vi "Burning2.1.vi"() -> ()   [LabVIEW 2022 SP3]
uses:
  Loop Handler/Main/Type Def/MainStates Cluster.ctl
  Loop Handler/Main/Type Def/MainStates.ctl
panel:
  out "Cartucho 8":dbl(graph)
  out "Cartucho 7":dbl(graph)
  out "Cartucho 6":dbl(graph)
  out "Cartucho 5":dbl(graph)
  out "Cartucho 4":dbl(graph)
  out "Cartucho 3":dbl(graph)
  out "Cartucho 2":dbl(graph)
  out "Cartucho 1":dbl(graph)
  out "0":cluster{i32, i32, i32, i32, i32, i32, i32, i32}={0, 1, 4, 5, 6, 7, 2, 3}
  out "Array":dbl[](array[numeric])
  in  "Cluster":T1
  in  "Prueba C":T2
  in  "SettingsCluster":T3={"OK Button Settings"=FALSE, "Default Set"=FALSE, "D Turbine"=FALSE, "D Panel"=FALSE, "D Date"=FALSE, "Delete Results"=FALSE, "file"=path "D:/config.ini"}
  out "Done":bool
  out "Start Time":string
  out "End Time":string
  out "Current Time":string
  out "Tmin":dbl
  out "Tmax":dbl
  out "CoolD":dbl
  out "TestT":dbl
  out "Contra":string
  out "values":string[](array[string])
  in  "Stop Test":bool
  in  "Start Test":bool
  in  "String 2":string
  out "Boolean":bool
  out "Numeric 2":dbl
  out "Array 3":string[](array[string])
  in  "Part Number":string
  in  "Help":bool
  out "EMO":bool
  in  "Cartuchos":u32[](array[colorbox]) caption="Cartridges"
  in  "Settings":bool
  in  "Results":bool
  in  "U settings":bool
  in  "Exit Button":bool
  in  "Lenguage":bool
  in  "Sets":T4
  out "offset past number":i32
  out "number":dbl
  out "data out":string
  out "bytes written":i32
  out "Numeric":dbl
  out "date/time string":string
  out "Acción":string
  out "Voltaje de salida":dbl caption="Output Voltage"
  in  "Voltage":bool
  in  "Probes":bool
  out "No. T":dbl caption="No. of Tests"
  out "Indicators":T5={"Error Out Array"=[], "Modbus"=FALSE, "Enet"=FALSE, "Ready"=FALSE, "Voltage output"=FALSE, "Prueba"=TRUE}
  # "MSE"
  # "1"
  # "2"
  # "3"
  # "4"
  # "5"
  # "6"
  # "7"
  # "8"
  # "DC Voltage"
  # "AC Voltage"
  # "Test"
  # "SETTINGS"
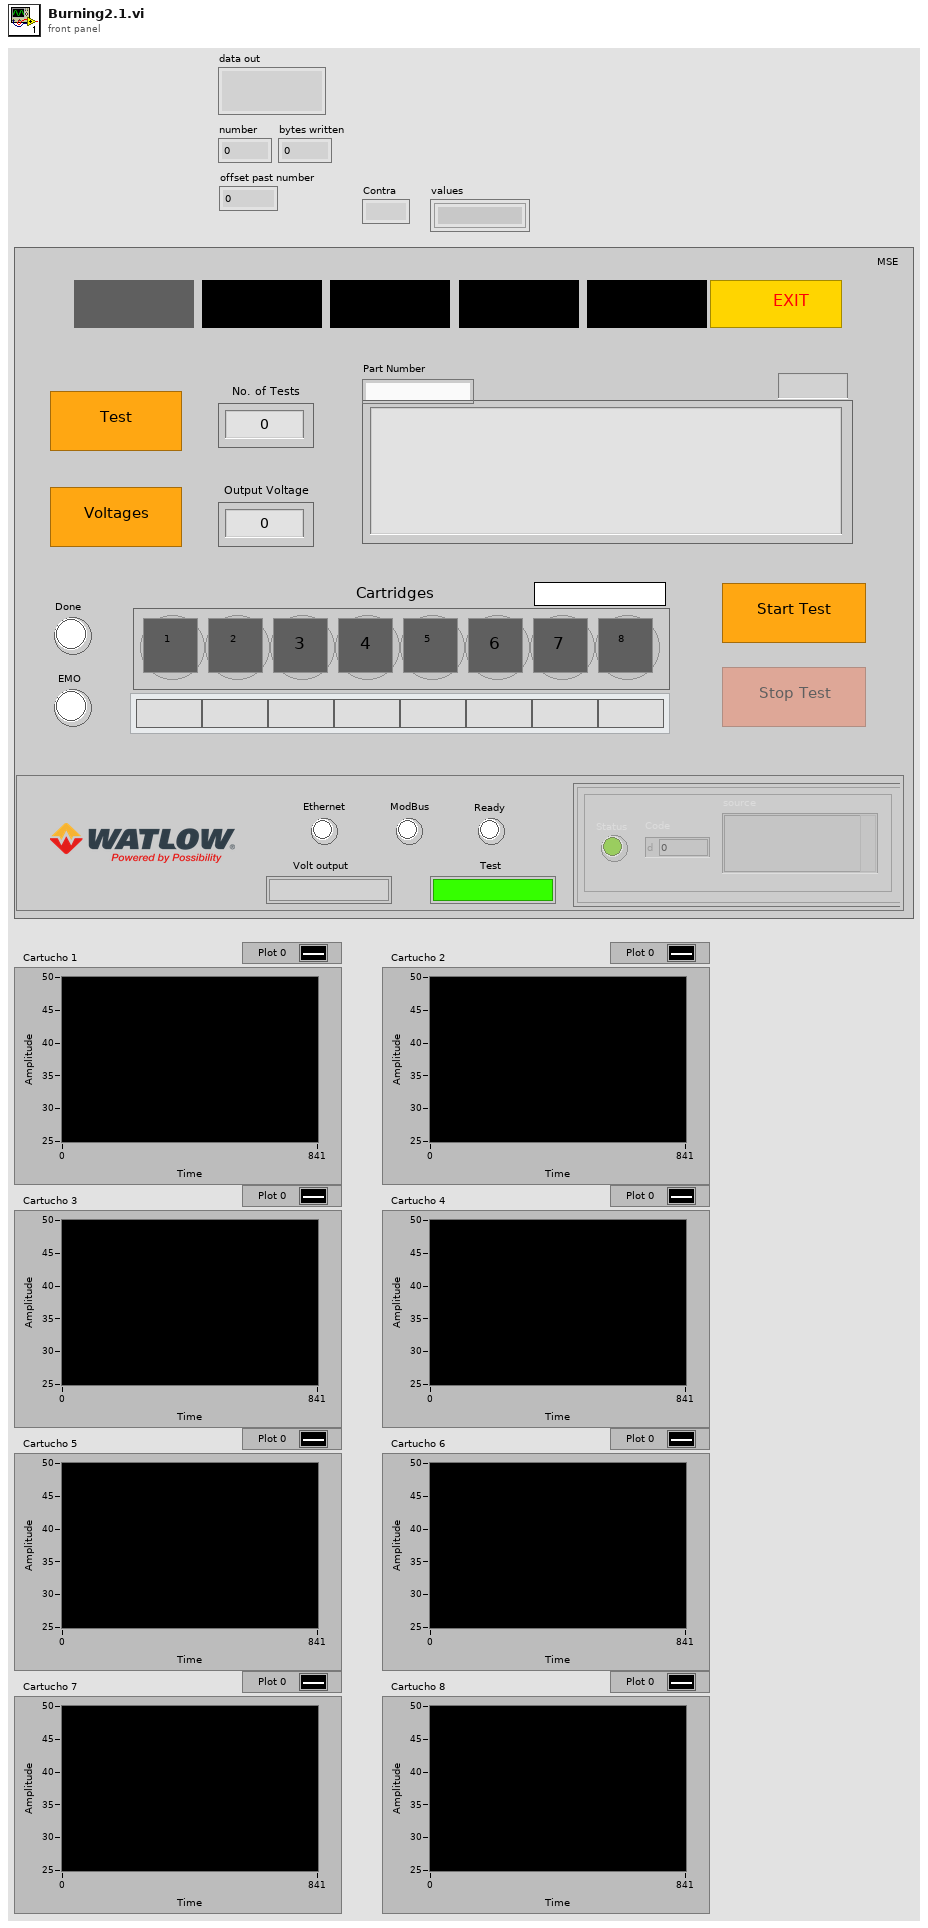
[diagram p1: front panel]
types:
  T1 = cluster{"24v":bool, "48v":bool, "110v":bool, "220v":bool, "OK Button Volts":bool, "Cancel Button Volts":bool}
  T2 = cluster{"OK Button":bool, "Tiempo Prueba":dbl, "Tiempo enfriamiento":dbl, "Temp- Max":dbl, "Tempo - Min":dbl, "Default Test":bool, "Cancel Button Test":bool}
  T3 = cluster{"OK Button Settings":bool, "Default Set":bool, "D Turbine":bool, "D Panel":bool, "D Date":bool, "Delete Results":bool, "file":path}
  T4 = cluster{"String":string, "String 2":string, "String 3":string, "String 4":string}
  T5 = cluster{"Error Out Array":errorcluster[], "Modbus":bool, "Enet":bool, "Ready":bool, "Voltage output":bool, "Prueba":bool}
  T6 = typedef "MainStates Cluster.ctl" = cluster{"States":T7, "Data":variant}
  T7 = typedef "MainStates.ctl" = enum16{"Open Ports", "Set_Config", "Close Ports", "Main", "Settings", "Volts", "Lenguaje", "Test", "End test", "EMO", "Exit"}
  T8 = cluster{"Error Out Array":errorcluster[], "34970A":bool, "53220A":bool, "USB-CAN":bool, "USB-LIN":bool, "Voltage output":bool}
  T9 = enum8{"Enabled", "Disabled", "Disabled and Grayed Out"}
  T10 = enum16{"Standard", "Buffered", "CRLF", "Immediate"}
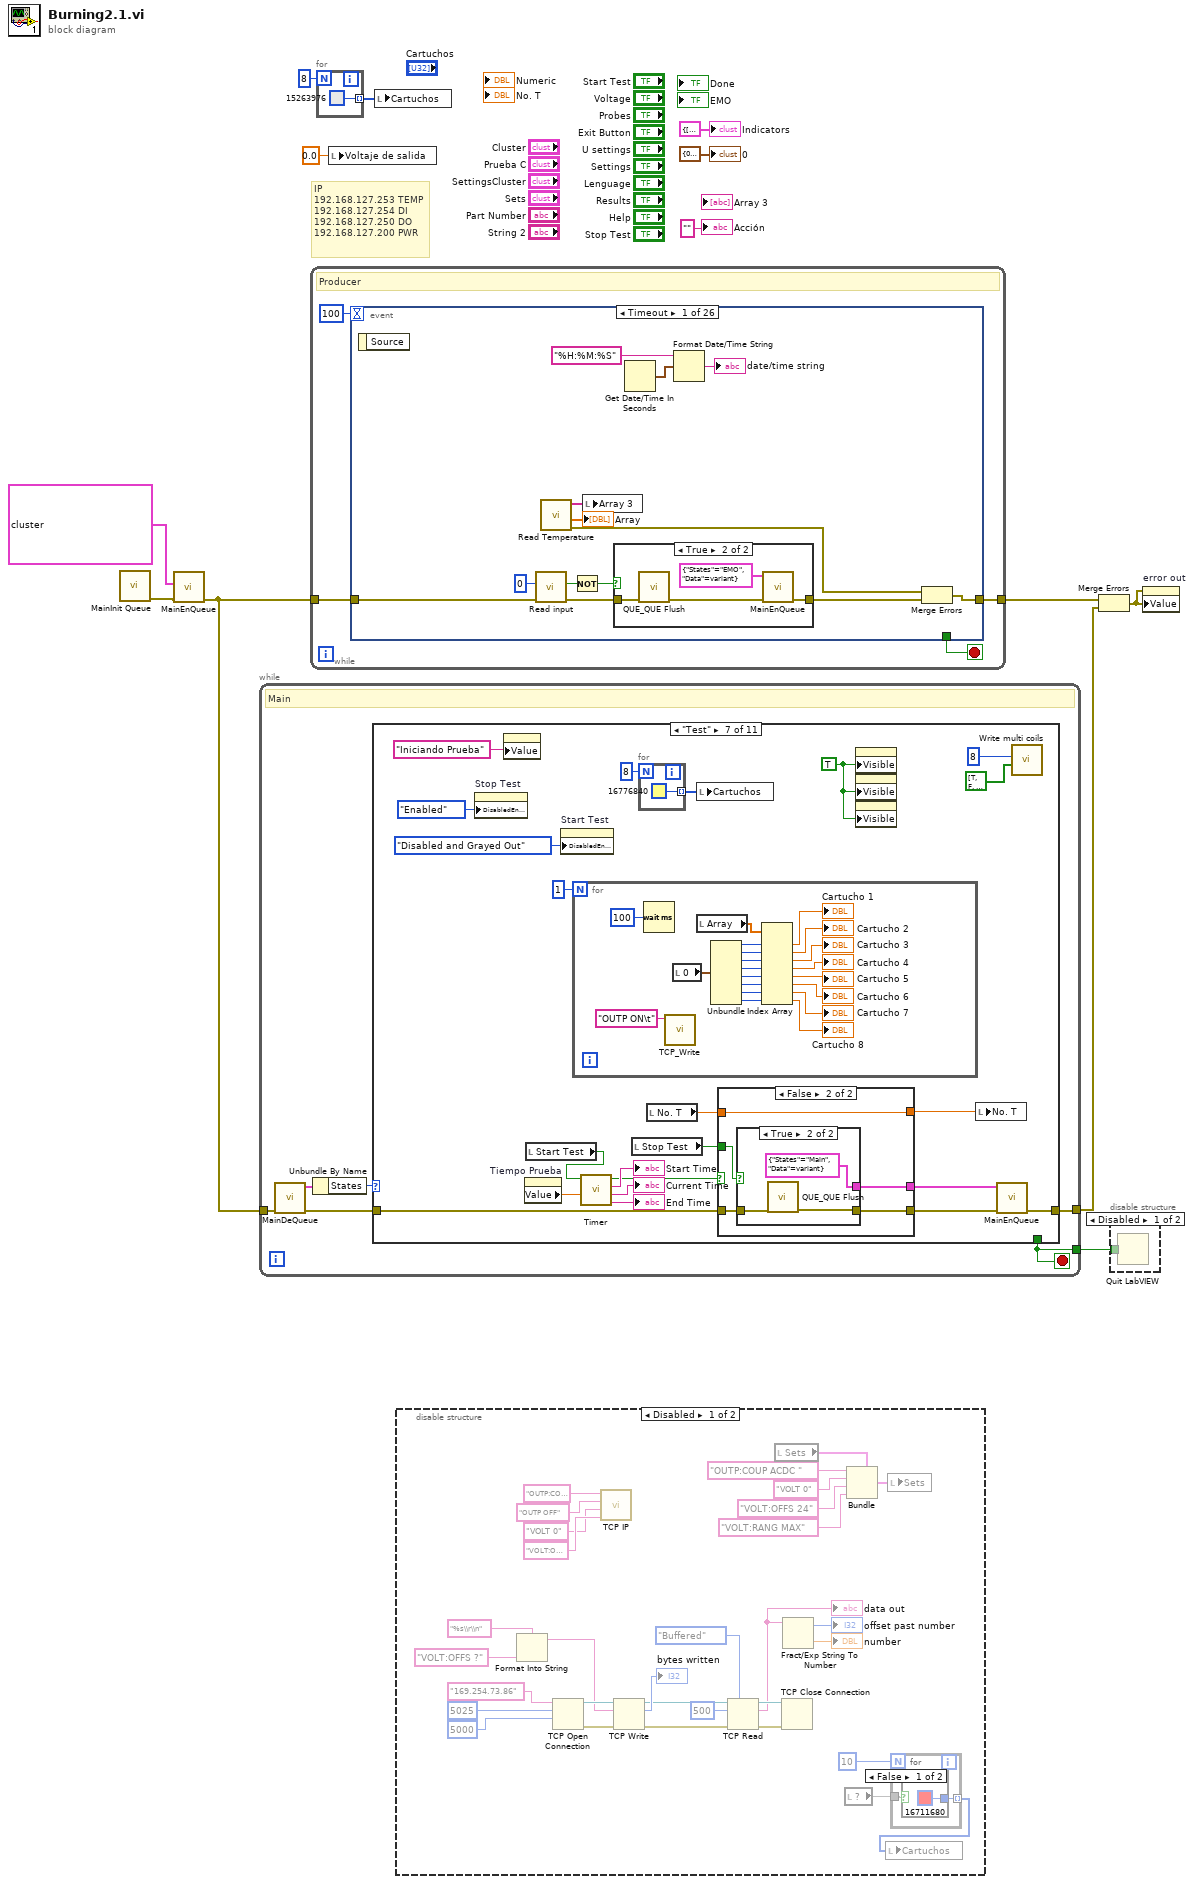
[diagram p0: block diagram]
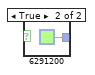
[diagram p2: hidden frame]
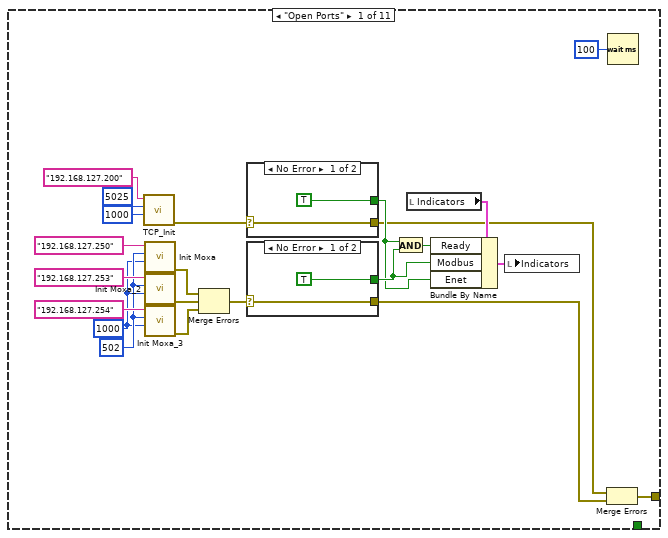
[diagram p5: hidden frame]
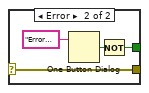
[diagram p6: hidden frame]
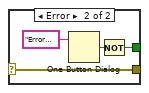
[diagram p7: hidden frame]
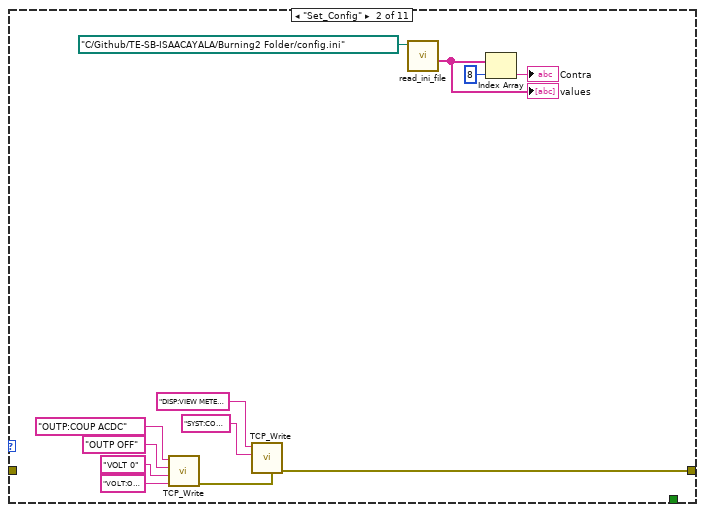
[diagram p8: hidden frame]
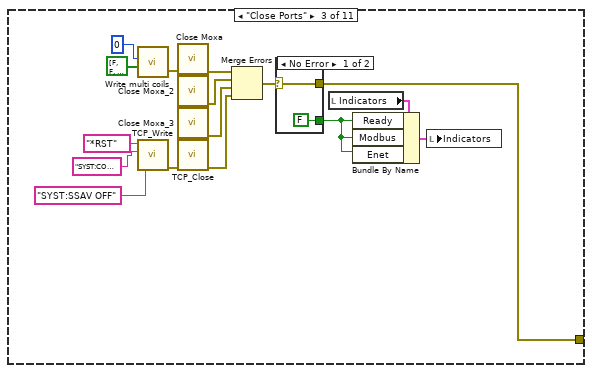
[diagram p9: hidden frame]
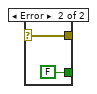
[diagram p10: hidden frame]
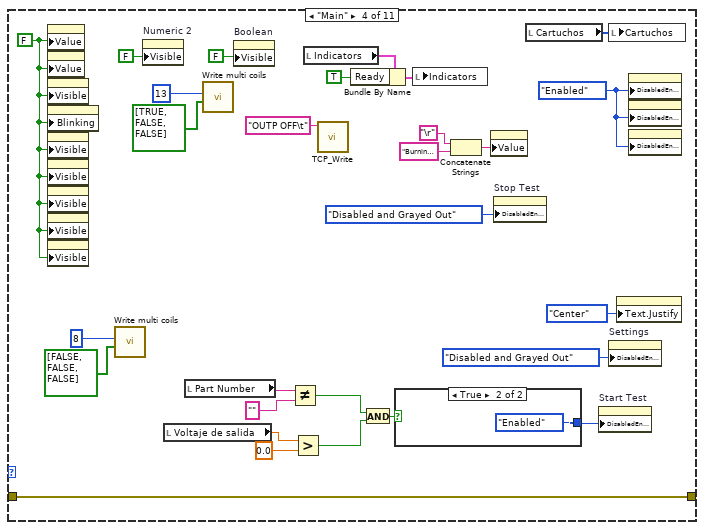
[diagram p11: hidden frame]
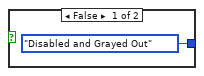
[diagram p12: hidden frame]
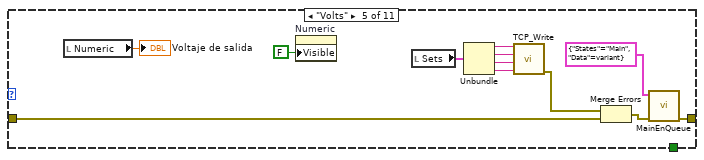
[diagram p13: hidden frame]
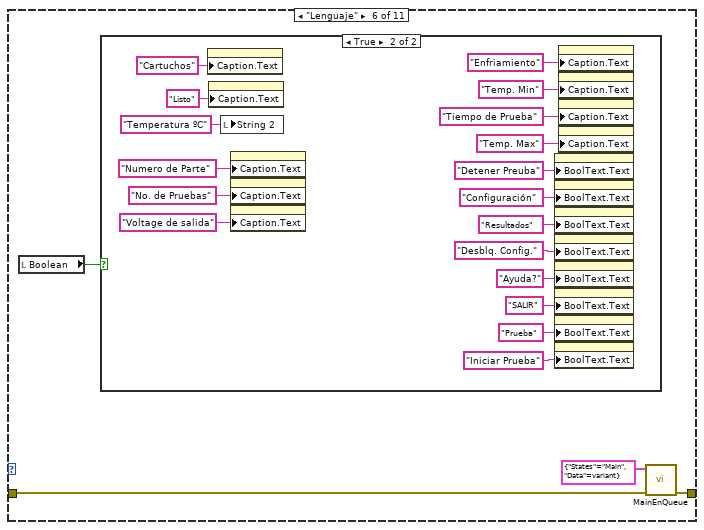
[diagram p14: hidden frame]
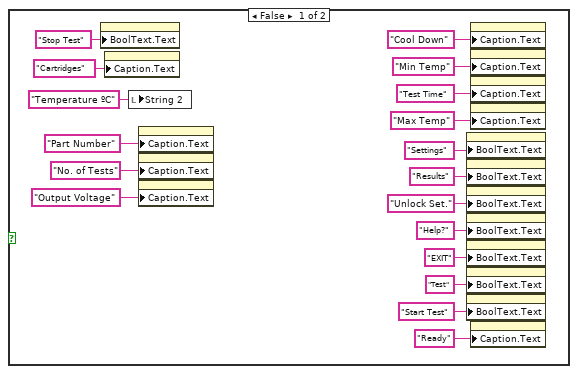
[diagram p15: hidden frame]
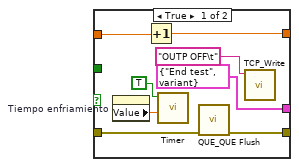
[diagram p16: hidden frame]
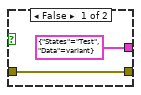
[diagram p17: hidden frame]
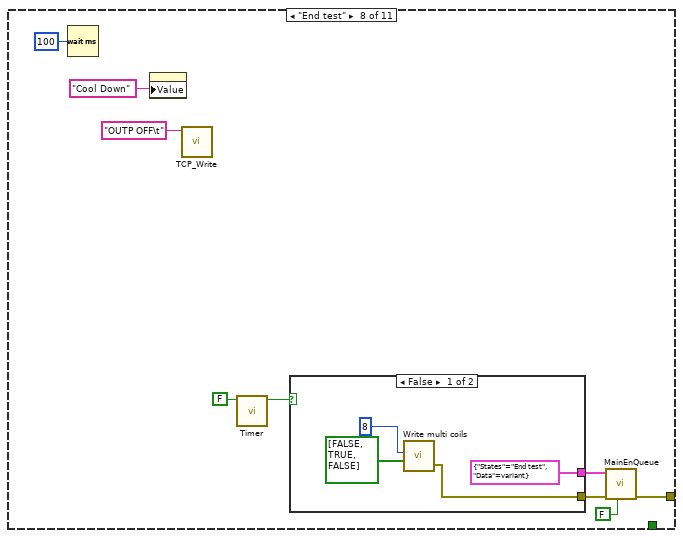
[diagram p18: hidden frame]
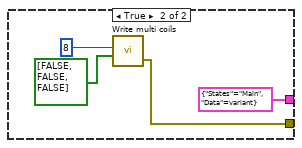
[diagram p19: hidden frame]
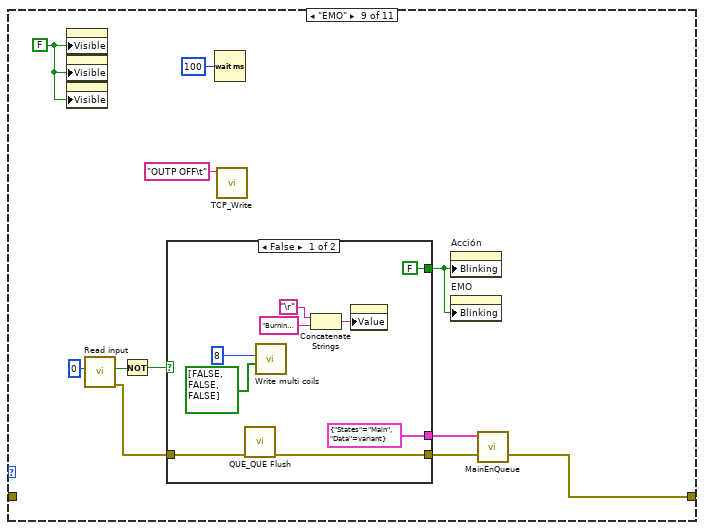
[diagram p20: hidden frame]
diagram:
  # "IP\n192.168.127.253 TEMP\n192.168.127.254 DI\n192.168.127.250 DO \n192.168.127.200 PWR"
  n1 = call "MainInit Queue.vi"() -> ("error out"=w11:errorcluster)  [unwired: 11 in]
  n2 = call "MainEnQueue.vi"("error in"=w11, "Array States"=T6[] [{"States"=enum."Open Ports", "Data"=variant}, {"States"=enum."Set_Config", "Data"=variant}, {"States"=enum."Main", "Data"=variant}]) -> ("error out"=w10:errorcluster)  [unwired: 9 in]
  n3 = while {
    tunnel: [w19] -> w8
    tunnel: [w18] -> w13
    tunnel: w10 -> [w16]
    stop <- w18 stop-if-true
    # "Main"
    n4 = call "MainDeQueue.vi"("error in"=w16) -> ("error out"=w15:errorcluster, "States"=w17:T6)  [unwired: 8 in, 1 out]
    n5 = Unbundle By Name(w17) -> ("States"=w14:T7)
    n6 = case shown="\"Test\"" w14 {
      tunnel: [_ _ _ _ _ _ _ _ _ TRUE _] -> w18
      tunnel: [w22 w58 w74 w90 w127 w131 w172 w237 w252 w276 _] -> w19
      tunnel: w15 -> [_ _ _ w90 w118 w128 w175 _ _ _ _]
      frame "Open Ports" {
        w30 = 1000 ("connect timeout ms")
        w31 = u16 502 ("port")
        n7 = call "TCP_Init.vi"("timeout ms (60000)"=1000, "remote port or service name"=u16 5025, "address"="192.168.127.200") -> ("error out 2"=w26:errorcluster)  [unwired: 6 in, 2 out]
        n8 = call "Init Moxa.vi"("connect timeout ms"=w30, "port"=w31, "Address"="192.168.127.250") -> ("error out"=w34:errorcluster)  [unwired: 6 in, 2 out]
        n9 = call "Init Moxa_2.vi"("connect timeout ms"=w30, "port"=w31, "Address"="192.168.127.253") -> ("error out"=w33:errorcluster)  [unwired: 6 in, 2 out]
        n10 = call "Init Moxa_3.vi"("connect timeout ms"=w30, "port"=w31, "Address"="192.168.127.254") -> ("error out"=w32:errorcluster)  [unwired: 6 in, 2 out]
        n11 = Merge Errors(w34, w33, w32) -> (w41:errorcluster)
        n12 = case shown="No Error" w26 {
          selector: w26 -> [w43 w46]
          tunnel: [w43 w46] -> w21
          tunnel: [TRUE ("true") w45] -> w23
          frame No Error {
          }
          frame Error {
            n13 = One Button Dialog(message="Error Power Supply") -> (true=w44:bool)  [unwired: 1 in]
            n14 = Not(x=w44) -> (.not. x?=w45:bool)
          }
        }
        n15 = case shown="No Error" w41 {
          selector: w41 -> [w49 w52]
          tunnel: [w49 w52] -> w20
          tunnel: [TRUE ("true") w51] -> w24
          frame No Error {
          }
          frame Error {
            n16 = One Button Dialog(message="Error Moxas") -> (true=w50:bool)  [unwired: 1 in]
            n17 = Not(x=w50) -> (.not. x?=w51:bool)
          }
        }
        n18 = And(x=w23, y=w24) -> (x .and. y?=w25:bool)
        n19 = local read "Indicators"() -> (w40:T5)
        n20 = Bundle By Name(cluster=w40, "Ready"=w25, "Modbus"=w24, "Enet"=w23) -> (w39:T5)
        n21 = local write "Indicators"(w39) -> ()
        n22 = Merge Errors(w21, w20) -> (w22:errorcluster)
        n23 = Wait (ms)(milliseconds to wait=u32 100) -> ()  [unwired: 1 out]
      }
      frame "Set_Config" {
        n24 = call "TCP_Write.vi"("String 1"="OUTP:COUP ACDC", "String 4"="OUTP OFF" ("String 2"), "String 3"="VOLT 0", "String 2"="VOLT:OFFS 0" ("String 4")) -> ("error out"=w61:errorcluster)  [unwired: 4 in, 1 out]
        n25 = call "TCP_Write.vi"("String 1"="DISP:VIEW METER_VI\n", "String 4"="SYST:COMM:RLST RWL", "error in (no error) 2"=w61) -> ("error out"=w58:errorcluster)  [unwired: 5 in, 1 out]
        n26 = call "read_ini_file.vi"("configuration file path"=path "C:/Github/TE-SB-ISAACAYALA/Burning2 Folder/config.ini") -> ("values"=w56:string[])  [unwired: 7 in, 3 out]
        "values" <- w56
        n27 = Index Array(array=w56, index=8) -> (element=→"Contra":string)
      }
      frame "Close Ports" {
        n28 = call "Write multi coils.vi"("coils to write"=bool[] [FALSE, FALSE, FALSE, FALSE, FALSE, FALSE, FALSE, FALSE, FALSE, FALSE, FALSE, FALSE, FALSE, FALSE, FALSE], "starting address"=u16 0) -> ("error IO"=w71:errorcluster)  [unwired: 2 in, 1 out]
        n29 = call "TCP_Write.vi"("String 1"="*RST", "String 4"="SYST:COMM:RLST LOC", "String 3"="SYST:SSAV OFF") -> ("error out"=w68:errorcluster)  [unwired: 5 in, 1 out]
        n30 = call "Close Moxa.vi"("error in (no error)"=w71) -> ("error out"=w79:errorcluster)  [unwired: 10 in]
        n31 = call "Close Moxa_2.vi"() -> ("error out"=w80:errorcluster)  [unwired: 11 in]
        n32 = call "Close Moxa_3.vi"() -> ("error out"=w81:errorcluster)  [unwired: 11 in]
        n33 = call "TCP_Close.vi"("error in (no error) 2"=w68) -> ("error out"=w70:errorcluster)  [unwired: 10 in]
        n34 = Merge Errors(w79, w80, w81, w70) -> (w76:errorcluster)
        n35 = case shown="No Error" w76 {
          selector: w76 -> [w82 w85]
          tunnel: [FALSE ("Enet") FALSE ("Enet")] -> w75
          tunnel: [w82 w85] -> w74
          frame No Error {
          }
          frame Error {
          }
        }
        n36 = local read "Indicators"() -> (w78:T5)
        n37 = Bundle By Name(cluster=w78, "Ready"=w75, "Modbus"=w75, "Enet"=w75) -> (w77:T5)
        n38 = local write "Indicators"(w77) -> ()
      }
      frame "Main" {
        w87 = FALSE ("Value")
        w107 = T9."Enabled" ("Disabled")
        n39 = property on="Prueba" class="Bool (strict)"("Value"=w87) -> ()  [unwired: 2 in, 2 out]
        n40 = property on="Voltage output" class="Bool (strict)"("Value"=w87) -> ()  [unwired: 2 in, 2 out]
        n41 = property on="SettingsCluster" class="Clust (strict)"("Visible"=w87) -> ()  [unwired: 2 in, 2 out]
        n42 = property on="Acción" class="Str"("Blinking"=w87) -> ()  [unwired: 2 in, 2 out]
        n43 = property on="Cluster" class="Clust (strict)"("Visible"=w87) -> ()  [unwired: 2 in, 2 out]
        n44 = property on="Prueba C" class="Clust (strict)"("Visible"=w87) -> ()  [unwired: 2 in, 2 out]
        n45 = property on="Start Time" class="Str"("Visible"=w87) -> ()  [unwired: 2 in, 2 out]
        n46 = property on="End Time" class="Str"("Visible"=w87) -> ()  [unwired: 2 in, 2 out]
        n47 = property on="Current Time" class="Str"("Visible"=w87) -> ()  [unwired: 2 in, 2 out]
        n48 = call "Write multi coils.vi"("coils to write"=bool[] [FALSE, FALSE, FALSE], "starting address"=u16 8) -> ()  [unwired: 2 in, 2 out]
        n49 = property on="Numeric 2" class="DigNum (strict)"("Visible"=FALSE) -> ()  [unwired: 2 in, 2 out]
        n50 = local read "Voltaje de salida"() -> (w100:dbl)
        n51 = local read "Part Number"() -> (w98:string)
        n52 = call "Write multi coils.vi"("coils to write"=bool[] [TRUE, FALSE, FALSE], "starting address"=u16 13) -> ()  [unwired: 2 in, 2 out]
        n53 = property on="Boolean" class="Bool (strict)"("Visible"=FALSE) -> ()  [unwired: 2 in, 2 out]
        n54 = Not Equal?(x=w98, y="") -> (x != y?=w95:bool)
        n55 = Greater?(x=w100, y=0.0 ("x")) -> (0:w96:bool)
        n56 = local read "Indicators"() -> (w111:T5)
        n57 = call "TCP_Write.vi"("String 1"="OUTP OFF\t") -> ()  [unwired: 7 in, 2 out]
        n58 = Bundle By Name(cluster=w111, "Ready"=TRUE) -> (w110:T5)
        n59 = And(x=w95, y=w96) -> (x .and. y?=w94:bool)
        n60 = case shown="True" w94 {
          tunnel: [T9."Disabled and Grayed Out" ("Disabled") T9."Enabled" ("Disabled")] -> w101
          frame False {
          }
          frame True {
          }
        }
        n61 = local write "Indicators"(w110) -> ()
        n62 = Concatenate Strings("\r" ("Carriage Return Constant"), "Burning Tester 1.1" ("Acción")) -> (w106:string)
        n63 = property on="Acción" class="Str"("Value"=w106) -> ()  [unwired: 2 in, 2 out]
        n64 = property on="Stop Test" class="Bool (strict)"("DisabledEnum"=T9."Disabled and Grayed Out" ("Disabled")) -> ()  [unwired: 2 in, 2 out]
        n65 = local read "Cartuchos"() -> (w113:u32[])
        n66 = property on="Start Test" class="Bool (strict)"("DisabledEnum"=w101) -> ()  [unwired: 2 in, 2 out]
        n67 = local write "Cartuchos"(w113) -> ()
        n68 = property on="Settings" class="Bool (strict)"("DisabledEnum"=T9."Disabled and Grayed Out" ("Disabled")) -> ()  [unwired: 2 in, 2 out]
        n69 = property on="Acción" class="Str"("Text.Justify"=enum16{"Left", "Center", "Right"}."Center" ("Text.Justification")) -> ()  [unwired: 2 in, 2 out]
        n70 = property on="Voltage" class="Bool (strict)"("DisabledEnum"=w107) -> ()  [unwired: 2 in, 2 out]
        n71 = property on="Probes" class="Bool (strict)"("DisabledEnum"=w107) -> ()  [unwired: 2 in, 2 out]
        n72 = property on="U settings" class="Bool (strict)"("DisabledEnum"=w107) -> ()  [unwired: 2 in, 2 out]
      }
      frame "Volts" {
        n73 = local read "Numeric"() -> (→"Voltaje de salida":dbl)
        n74 = property on="Numeric" class="DigNum (strict)"("Visible"=FALSE) -> ()  [unwired: 2 in, 2 out]
        n75 = local read "Sets"() -> (w124:T4)
        n76 = Unbundle(w124) -> ("String"=w122:string, "String 2"=w121:string, "String 3"=w120:string, "String 4"=w119:string)
        n77 = call "TCP_Write.vi"("String 1"=w122, "String 4"=w121, "String 3"=w120, "String 2"=w119) -> ("error out"=w117:errorcluster)  [unwired: 4 in, 1 out]
        n78 = Merge Errors(w117, w118) -> (w116:errorcluster)
        n79 = call "MainEnQueue.vi"("error in"=w116, "States"=T6 {"States"=enum."Main", "Data"=variant}) -> ("error out"=w127:errorcluster)  [unwired: 9 in]
      }
      frame "Lenguaje" {
        n80 = local read "Boolean"() -> (w129:bool)
        n81 = case shown="True" w129 {
          frame False {
            n82 = property on="Stop Test" class="Bool (strict)"("BoolText.Text"="Stop Test" ("Boolean Text.Text")) -> ()  [unwired: 2 in, 2 out]
            n83 = property on="Cartuchos" class="Arr (strict)"("Caption.Text"="Cartridges") -> ()  [unwired: 2 in, 2 out]
            n84 = local write "String 2"("Temperature ºC" ("String 2")) -> ()
            n85 = property on="Part Number" class="Str"("Caption.Text"="Part Number") -> ()  [unwired: 2 in, 2 out]
            n86 = property on="No. T" class="DigNum (strict)"("Caption.Text"="No. of Tests") -> ()  [unwired: 2 in, 2 out]
            n87 = property on="Voltaje de salida" class="DigNum (strict)"("Caption.Text"="Output Voltage") -> ()  [unwired: 2 in, 2 out]
            n88 = property on="Settings" class="Bool (strict)"("BoolText.Text"="Settings" ("Boolean Text.Text")) -> ()  [unwired: 2 in, 2 out]
            n89 = property on="Results" class="Bool (strict)"("BoolText.Text"="Results" ("Boolean Text.Text")) -> ()  [unwired: 2 in, 2 out]
            n90 = property on="U settings" class="Bool (strict)"("BoolText.Text"="Unlock Set." ("Boolean Text.Text")) -> ()  [unwired: 2 in, 2 out]
            n91 = property on="Help" class="Bool (strict)"("BoolText.Text"="Help?" ("Boolean Text.Text")) -> ()  [unwired: 2 in, 2 out]
            n92 = property on="Exit Button" class="Bool (strict)"("BoolText.Text"="EXIT" ("Boolean Text.Text")) -> ()  [unwired: 2 in, 2 out]
            n93 = property on="Probes" class="Bool (strict)"("BoolText.Text"="Test" ("Boolean Text.Text")) -> ()  [unwired: 2 in, 2 out]
            n94 = property on="Start Test" class="Bool (strict)"("BoolText.Text"="Start Test" ("Boolean Text.Text")) -> ()  [unwired: 2 in, 2 out]
            n95 = property on="Tiempo enfriamiento" class="DigNum (strict)"("Caption.Text"="Cool Down") -> ()  [unwired: 2 in, 2 out]
            n96 = property on="Tempo - Min" class="DigNum (strict)"("Caption.Text"="Min Temp") -> ()  [unwired: 2 in, 2 out]
            n97 = property on="Tiempo Prueba" class="DigNum (strict)"("Caption.Text"="Test Time") -> ()  [unwired: 2 in, 2 out]
            n98 = property on="Temp- Max" class="DigNum (strict)"("Caption.Text"="Max Temp") -> ()  [unwired: 2 in, 2 out]
            n99 = property on="Ready" class="Bool (strict)"("Caption.Text"="Ready") -> ()  [unwired: 2 in, 2 out]
          }
          frame True {
            n100 = property on="Cartuchos" class="Arr (strict)"("Caption.Text"="Cartuchos") -> ()  [unwired: 2 in, 2 out]
            n101 = property on="Ready" class="Bool (strict)"("Caption.Text"="Listo") -> ()  [unwired: 2 in, 2 out]
            n102 = local write "String 2"("Temperatura ºC" ("String 2")) -> ()
            n103 = property on="Part Number" class="Str"("Caption.Text"="Numero de Parte") -> ()  [unwired: 2 in, 2 out]
            n104 = property on="No. T" class="DigNum (strict)"("Caption.Text"="No. de Pruebas") -> ()  [unwired: 2 in, 2 out]
            n105 = property on="Voltaje de salida" class="DigNum (strict)"("Caption.Text"="Voltage de salida") -> ()  [unwired: 2 in, 2 out]
            n106 = property on="Stop Test" class="Bool (strict)"("BoolText.Text"="Detener Preuba" ("Boolean Text.Text")) -> ()  [unwired: 2 in, 2 out]
            n107 = property on="Settings" class="Bool (strict)"("BoolText.Text"="Configuración" ("Boolean Text.Text")) -> ()  [unwired: 2 in, 2 out]
            n108 = property on="Results" class="Bool (strict)"("BoolText.Text"="Resultados" ("Boolean Text.Text")) -> ()  [unwired: 2 in, 2 out]
            n109 = property on="U settings" class="Bool (strict)"("BoolText.Text"="Desblq. Config." ("Boolean Text.Text")) -> ()  [unwired: 2 in, 2 out]
            n110 = property on="Help" class="Bool (strict)"("BoolText.Text"="Ayuda?" ("Boolean Text.Text")) -> ()  [unwired: 2 in, 2 out]
            n111 = property on="Exit Button" class="Bool (strict)"("BoolText.Text"="SALIR" ("Boolean Text.Text")) -> ()  [unwired: 2 in, 2 out]
            n112 = property on="Probes" class="Bool (strict)"("BoolText.Text"="Prueba" ("Boolean Text.Text")) -> ()  [unwired: 2 in, 2 out]
            n113 = property on="Start Test" class="Bool (strict)"("BoolText.Text"="Iniciar Prueba" ("Boolean Text.Text")) -> ()  [unwired: 2 in, 2 out]
            n114 = property on="Tiempo enfriamiento" class="DigNum (strict)"("Caption.Text"="Enfriamiento") -> ()  [unwired: 2 in, 2 out]
            n115 = property on="Tempo - Min" class="DigNum (strict)"("Caption.Text"="Temp. Min") -> ()  [unwired: 2 in, 2 out]
            n116 = property on="Tiempo Prueba" class="DigNum (strict)"("Caption.Text"="Tiempo de Prueba") -> ()  [unwired: 2 in, 2 out]
            n117 = property on="Temp- Max" class="DigNum (strict)"("Caption.Text"="Temp. Max") -> ()  [unwired: 2 in, 2 out]
          }
        }
        n118 = call "MainEnQueue.vi"("error in"=w128, "States"=T6 {"States"=enum."Main", "Data"=variant}) -> ("error out"=w131:errorcluster)  [unwired: 9 in]
      }
      frame "Test" {
        w188 = TRUE ("Visible")
        n119 = property on="Stop Test" class="Bool (strict)"("DisabledEnum"=T9."Enabled" ("Disabled")) -> ()  [unwired: 2 in, 2 out]
        n120 = property on="Acción" class="Str"("Value"="Iniciando Prueba" ("Acción")) -> ()  [unwired: 2 in, 2 out]
        n121 = property on="Tiempo Prueba" class="DigNum (strict)"() -> ("Value"=w182:dbl)  [unwired: 2 in, 2 out]
        n122 = local read "Start Test"() -> (w183:bool)
        n123 = property on="Start Test" class="Bool (strict)"("DisabledEnum"=T9."Disabled and Grayed Out" ("Disabled")) -> ()  [unwired: 2 in, 2 out]
        n124 = for {
          N: 1 -> [_]
          n125 = Wait (ms)(milliseconds to wait=u32 100) -> ()  [unwired: 1 out]
          n126 = call "TCP_Write.vi"("String 1"="OUTP ON\t") -> ()  [unwired: 7 in, 2 out]
          n127 = local read "0"() -> (w208:cluster{i32, i32, i32, i32, i32, i32, i32, i32})
          n128 = local read "Array"() -> (w209:dbl[])
          n129 = Unbundle(w208) -> (w207:i32, w206:i32, w205:i32, w204:i32, w203:i32, w202:i32, w201:i32, w200:i32)
          n130 = Index Array(array=w209, index #1=w207, index #2=w206, index #3=w205, index #4=w204, index #5=w203, index #6=w202, index #7=w201, index #8=w200) -> (element #1=→"Cartucho 1":dbl, element #2=→"Cartucho 2":dbl, element #3=→"Cartucho 3":dbl, element #4=→"Cartucho 4":dbl, element #5=→"Cartucho 5":dbl, element #6=→"Cartucho 6":dbl, element #7=→"Cartucho 7":dbl, element #8=→"Cartucho 8":dbl)
        }
        n131 = call "Timer.vi"("Delay (sec)"=w182, "Reset timer"=w183) -> ("End Time"=→"End Time":string, "Current Time"=→"Current Time":string, "Start Time"=→"Start Time":string, "Time Elapsed"=w176:bool)  [unwired: 6 in]
        n132 = local read "Stop Test"() -> (w171:bool)
        n133 = for {
          N: 8 -> [_]
          tunnel: [u32 16776840] -> w184 mode=indexing
        }
        n134 = local read "No. T"() -> (w170:dbl)
        n135 = local write "Cartuchos"(w184) -> ()
        n136 = case shown="False" w176 {
          tunnel: w175 -> [w217 w220]
          tunnel: [w214 w219] -> w174
          tunnel: [T6 {"States"=enum."End test", "Data"=variant} ("States") w222] -> w173
          tunnel: w171 -> [_ w221]
          tunnel: w170 -> [w212 w218]
          tunnel: [w211 w218] -> w169
          frame True {
            n137 = property on="Tiempo enfriamiento" class="DigNum (strict)"() -> ("Value"=w216:dbl)  [unwired: 2 in, 2 out]
            n138 = Increment(x=w212) -> (x+1=w211:dbl)
            n139 = call "Timer.vi"("Delay (sec)"=w216, "Reset timer"=TRUE) -> ()  [unwired: 6 in, 4 out]
            n140 = call "QUE_QUE Flush.vi"("Error"=w217) -> ("Error Out"=w214:errorcluster)  [unwired: 10 in]
            n141 = call "TCP_Write.vi"("String 1"="OUTP OFF\t") -> ()  [unwired: 7 in, 2 out]
          }
          frame False {
            n142 = case shown="True" w221 {
              tunnel: [T6 {"States"=enum."Test", "Data"=variant} ("States") T6 {"States"=enum."Main", "Data"=variant} ("States")] -> w222
              tunnel: [w223 w225] -> w219
              tunnel: w220 -> [w223 w227]
              frame False {
              }
              frame True {
                n143 = call "QUE_QUE Flush.vi"("Error"=w227) -> ("Error Out"=w225:errorcluster)  [unwired: 10 in]
              }
            }
          }
        }
        n144 = property on="Start Time" class="Str"("Visible"=w188) -> ()  [unwired: 2 in, 2 out]
        n145 = property on="End Time" class="Str"("Visible"=w188) -> ()  [unwired: 2 in, 2 out]
        n146 = property on="Current Time" class="Str"("Visible"=w188) -> ()  [unwired: 2 in, 2 out]
        n147 = local write "No. T"(w169) -> ()
        n148 = call "MainEnQueue.vi"("error in"=w174, "States"=w173) -> ("error out"=w172:errorcluster)  [unwired: 9 in]
        n149 = call "Write multi coils.vi"("coils to write"=bool[] [TRUE, FALSE, FALSE, FALSE, FALSE, TRUE, TRUE], "starting address"=u16 8) -> ()  [unwired: 2 in, 2 out]
      }
      frame "End test" {
        n150 = Wait (ms)(milliseconds to wait=u32 100) -> ()  [unwired: 1 out]
        n151 = property on="Acción" class="Str"("Value"="Cool Down" ("Acción")) -> ()  [unwired: 2 in, 2 out]
        n152 = call "TCP_Write.vi"("String 1"="OUTP OFF\t") -> ()  [unwired: 7 in, 2 out]
        n153 = call "Timer.vi"("Reset timer"=FALSE) -> ("Time Elapsed"=w235:bool)  [unwired: 7 in, 3 out]
        n154 = case shown="False" w235 {
          tunnel: [T6 {"States"=enum."End test", "Data"=variant} ("States") T6 {"States"=enum."Main", "Data"=variant} ("States")] -> w236
          tunnel: [w238 w242] -> w234
          frame False {
            n155 = call "Write multi coils.vi"("coils to write"=bool[] [FALSE, TRUE, FALSE], "starting address"=u16 8) -> ("error IO"=w238:errorcluster)  [unwired: 2 in, 1 out]
          }
          frame True {
            n156 = call "Write multi coils.vi"("coils to write"=bool[] [FALSE, FALSE, FALSE], "starting address"=u16 8) -> ("error IO"=w242:errorcluster)  [unwired: 2 in, 1 out]
          }
        }
        n157 = call "MainEnQueue.vi"("Enqueue in Back?"=FALSE, "error in"=w234, "States"=w236) -> ("error out"=w237:errorcluster)  [unwired: 8 in]
      }
      frame "EMO" {
        w248 = FALSE ("Visible")
        n158 = property on="Start Time" class="Str"("Visible"=w248) -> ()  [unwired: 2 in, 2 out]
        n159 = property on="End Time" class="Str"("Visible"=w248) -> ()  [unwired: 2 in, 2 out]
        n160 = property on="Current Time" class="Str"("Visible"=w248) -> ()  [unwired: 2 in, 2 out]
        n161 = call "Read input.vi"("Input"=0) -> ("error out"=w251:errorcluster, "State"=w254:bool)  [unwired: 9 in]
        n162 = Not(x=w254) -> (.not. x?=w253:bool)
        n163 = case shown="False" w253 {
          tunnel: [w258 w275] -> w252
          tunnel: w251 -> [w259 w275]
          tunnel: [FALSE ("Blinking") TRUE ("Blinking")] -> w250
          tunnel: [T6 {"States"=enum."Main", "Data"=variant} ("States") T6 {"States"=enum."EMO", "Data"=variant} ("States")] -> w249
          frame False {
            n164 = call "QUE_QUE Flush.vi"("Error"=w259) -> ("Error Out"=w258:errorcluster)  [unwired: 10 in]
            n165 = call "Write multi coils.vi"("coils to write"=bool[] [FALSE, FALSE, FALSE], "starting address"=u16 8) -> ()  [unwired: 2 in, 2 out]
            n166 = Concatenate Strings("\r" ("Carriage Return Constant"), "Burning Tester 1.1" ("Acción")) -> (w264:string)
            n167 = property on="Acción" class="Str"("Value"=w264) -> ()  [unwired: 2 in, 2 out]
          }
          frame True {
            n168 = local read "Indicators"() -> (w266:T5)
            n169 = Bundle By Name(cluster=w266, "Ready"=FALSE) -> (w267:T5)
            n170 = Concatenate Strings("\r" ("Carriage Return Constant"), "Emergency Stop" ("Acción")) -> (w274:string)
            n171 = call "Write multi coils.vi"("coils to write"=bool[] [FALSE, TRUE, FALSE], "starting address"=u16 13 ("Coil")) -> ()  [unwired: 2 in, 2 out]
            n172 = property on="Acción" class="Str"("Value"=w274) -> ()  [unwired: 2 in, 2 out]
            n173 = local write "Indicators"(w267) -> ()
          }
        }
        n174 = Wait (ms)(milliseconds to wait=u32 100) -> ()  [unwired: 1 out]
        n175 = call "TCP_Write.vi"("String 1"="OUTP OFF\t") -> ()  [unwired: 7 in, 2 out]
        n176 = property on="Acción" class="Str"("Blinking"=w250) -> ()  [unwired: 2 in, 2 out]
        n177 = property on="EMO" class="Bool (strict)"("Blinking"=w250) -> ()  [unwired: 2 in, 2 out]
        n178 = call "MainEnQueue.vi"("States"=w249) -> ()  [unwired: 10 in, 1 out]
      }
      frame "Exit" {
        n179 = call "MainEnQueue.vi"() -> ("error out"=w276:errorcluster)  [unwired: 11 in]
      }
      frame "Settings" {
      }
    }
  }
  n180 = while {
    tunnel: [w280] -> w9
    tunnel: w10 -> [w278]
    stop <- w281 stop-if-true
    # "Producer"
    n181 = event shown="[0] Timeout" {
      selector: _ -> [_ _ _ _ _ _ _ _ _ _ _ _ _ _ _ _ _ _ _ _ _ _ _ _ _ _]
      dyn-events: _ -> [_ _ _ _ _ _ _ _ _ _ _ _ _ _ _ _ _ _ _ _ _ _ _ _ _ _]
      timeout: 100 -> [_ _ _ _ _ _ _ _ _ _ _ _ _ _ _ _ _ _ _ _ _ _ _ _ _ _]
      tunnel: [_ _ _ _ _ _ _ _ _ _ _ _ _ _ _ _ _ TRUE _ _ _ _ _ _ _ _] -> w281
      tunnel: [w283 w300 w310 w313 w326 w334 w336 w339 _ _ _ _ _ _ w345 w365 _ w370 w375 _ _ _ _ w416 w420 w424] -> w280
      tunnel: w278 -> [w286 w300 w310 w313 w326 w334 w336 _ _ _ _ _ _ _ w343 _ _ w369 w373 _ _ _ _ _ _ w423]
      event Timeout {
        n182 = event-data() -> ()  [unwired: 1 in, 1 out]
        n183 = call "Read input.vi"("error in (no error)"=w286, "Input"=0) -> ("error out"=w290:errorcluster, "State"=w289:bool)  [unwired: 8 in]
        n184 = call "Read Temperature.vi"() -> ("error IO"=w285:errorcluster, "Array"=→"Array":dbl[], "decimal integer string"=w287:string[])  [unwired: 9 in]
        n185 = Not(x=w289) -> (.not. x?=w291:bool)
        n186 = local write "Array 3"(w287) -> ()
        n187 = case shown="True" w291 {
          tunnel: w290 -> [w295 w296]
          tunnel: [w295 w298] -> w284
          frame False {
          }
          frame True {
            n188 = call "QUE_QUE Flush.vi"("Error"=w296) -> ("Error Out"=w297:errorcluster)  [unwired: 10 in]
            n189 = call "MainEnQueue.vi"("error in"=w297, "States"=T6 {"States"=enum."EMO", "Data"=variant}) -> ("error out"=w298:errorcluster)  [unwired: 9 in]
          }
        }
        n190 = Get Date/Time In Seconds() -> (seconds since 1Jan1904=w294:timestamp)
        n191 = Format Date/Time String(time format string (%c)="%H:%M:%S", seconds (now)=w294) -> (date/time string=→"date/time string":string)  [unwired: 1 out]
        n192 = Merge Errors(w285, w284) -> (w283:errorcluster)
      }
      event "Voltage": Value Change {
        n193 = event-data() -> ()  [unwired: 1 in, 1 out]
        n194 = Concatenate Strings("\r", "Select a voltage" ("Acción")) -> (w303:string)
        n195 = property on="Cluster" class="Clust (strict)"("Visible"=TRUE) -> ()  [unwired: 2 in, 2 out]
        n196 = property on="Acción" class="Str"("Value"=w303) -> ()  [unwired: 2 in, 2 out]
      }
      event "Probes": Value Change {
        n197 = event-data() -> ()  [unwired: 1 in, 1 out]
        n198 = local read "Prueba C"() -> (w309:T2)
        n199 = Unbundle(w309) -> ("Tiempo Prueba"=→"TestT":dbl, "Tiempo enfriamiento"=→"CoolD":dbl, "Temp- Max"=→"Tmax":dbl, "Tempo - Min"=→"Tmin":dbl)  [unwired: 3 out]
        n200 = property on="Prueba C" class="Clust (strict)"("Visible"=TRUE) -> ()  [unwired: 2 in, 2 out]
      }
      event "Prueba C.Default Test": Value Change {
        n201 = event-data() -> ()  [unwired: 1 in, 1 out]
        n202 = call "read_ini_file.vi"("configuration file path"=path "C:/Github/TE-SB-ISAACAYALA/Burning2 Folder/config.ini") -> ("values"=w323:string[])  [unwired: 7 in, 3 out]
        n203 = local read "Prueba C"() -> (w325:T2)
        n204 = Fract/Exp String To Number(string=w323) -> (number=w322:dbl[])  [unwired: 3 in, 1 out]
        n205 = Index Array(array=w322, index #1=0 ("index"), index #2=1 ("index"), index #3=2 ("index"), index #4=3 ("index")) -> (element #1=w321:dbl, element #2=w320:dbl, element #3=w319:dbl, element #4=w318:dbl)
        n206 = Bundle(cluster=w325, "Tiempo Prueba"=w321, "Tiempo enfriamiento"=w320, "Temp- Max"=w319, "Tempo - Min"=w318) -> (w324:T2)  [unwired: 3 in]
        n207 = local write "Prueba C"(w324) -> ()
      }
      event "Prueba C.Cancel Button Test": Value Change {
        n208 = event-data() -> ()  [unwired: 1 in, 1 out]
        n209 = local read "Prueba C"() -> (w333:T2)
        n210 = local read "TestT"() -> (w332:dbl)
        n211 = local read "CoolD"() -> (w331:dbl)
        n212 = local read "Tmax"() -> (w330:dbl)
        n213 = local read "Tmin"() -> (w329:dbl)
        n214 = Bundle(cluster=w333, "Tiempo Prueba"=w332, "Tiempo enfriamiento"=w331, "Temp- Max"=w330, "Tempo - Min"=w329) -> (w328:T2)  [unwired: 3 in]
        n215 = local write "Prueba C"(w328) -> ()
        n216 = property on="Prueba C" class="Clust (strict)"("Visible"=FALSE) -> ()  [unwired: 2 in, 2 out]
      }
      event "Prueba C.OK Button": Value Change {
        n217 = event-data() -> ()  [unwired: 1 in, 6 out]
        n218 = property on="Prueba C" class="Clust (strict)"("Visible"=FALSE) -> ()  [unwired: 2 in, 2 out]
      }
      event "Settings": Value Change {
        n219 = event-data() -> ()  [unwired: 1 in, 1 out]
        n220 = property on="Acción" class="Str"("Text.Justify"=enum16{"Left", "Center", "Right"}."Left" ("Text.Justification")) -> ()  [unwired: 2 in, 2 out]
        n221 = property on="SettingsCluster" class="Clust (strict)"("Visible"=TRUE) -> ()  [unwired: 2 in, 2 out]
      }
      event "SettingsCluster.OK Button Settings": Value Change {
        n222 = event-data() -> ()  [unwired: 1 in, 6 out]
        n223 = property on="Acción" class="Str"("Text.Justify"=enum16{"Left", "Center", "Right"}."Center" ("Text.Justification")) -> ()  [unwired: 2 in, 2 out]
        n224 = property on="SettingsCluster" class="Clust (strict)"("Visible"=FALSE) -> ()  [unwired: 2 in, 2 out]
        n225 = call "MainEnQueue.vi"("States"=T6 {"States"=enum."Main", "Data"=variant}) -> ("error out"=w339:errorcluster)  [unwired: 10 in]
      }
      event "SettingsCluster.Default Set": Value Change {
        n226 = event-data() -> ()  [unwired: 1 in, 6 out]
      }
      event "SettingsCluster.D Turbine": Value Change {
        n227 = event-data() -> ()  [unwired: 1 in, 6 out]
      }
      event "SettingsCluster.D Panel": Value Change {
        n228 = event-data() -> ()  [unwired: 1 in, 6 out]
      }
      event "SettingsCluster.D Date": Value Change {
        n229 = event-data() -> ()  [unwired: 1 in, 6 out]
      }
      event "SettingsCluster.Delete Results": Value Change {
        n230 = event-data() -> ()  [unwired: 1 in, 6 out]
      }
      event "Results": Value Change {
        n231 = event-data() -> ()  [unwired: 1 in, 6 out]
      }
      event "U settings": Value Change {
        n232 = event-data() -> ("NewVal"=w347:bool)  [unwired: 1 in]
        n233 = case shown="True" w347 {
          tunnel: [_ w353] -> w346
          tunnel: [errorcluster {"status"=FALSE, "code"=0, "source"=""} ("error out") w352] -> _
          frame False {
          }
          frame True {
            n234 = local read "Contra"() -> (w351:string)
            n235 = call "Prompt User for Input"("Enable"=TRUE) -> ("Password"=w354:string, "error out"=w352:errorcluster)  [unwired: 16 in, 1 out]
            n236 = Equal?(x=w351, y=w354) -> (x = y?=w353:bool)
          }
        }
        n237 = case shown="True" w346 {
          frame False {
          }
          frame True {
            n238 = property on="Settings" class="Bool (strict)"("DisabledEnum"=T9."Enabled" ("Disabled")) -> ()  [unwired: 2 in, 2 out]
            n239 = property on="U settings" class="Bool (strict)"("DisabledEnum"=T9."Disabled and Grayed Out" ("Disabled")) -> ()  [unwired: 2 in, 2 out]
          }
        }
        n240 = call "MainEnQueue.vi"("error in"=w343, "States"=T6 {"States"=enum."Settings", "Data"=variant}) -> ("error out"=w345:errorcluster)  [unwired: 9 in]
      }
      event "Lenguage": Value Change {
        n241 = event-data() -> ("NewVal"=w363:bool)  [unwired: 1 in]
        n242 = local read "Numeric 2"() -> (w361:dbl)
        n243 = Boolean To (0,1)(Boolean=w363) -> (0, 1=w362:i16)
        n244 = Add(x=w362, y=w361) -> (x+y=w359:dbl)
        "Numeric 2" <- w359
        n245 = Greater Or Equal?(x=w359, y=2.0) -> (x >= y?=w357:bool)
        n246 = Equal?(x=w359, y=1.0) -> (x = y?=w356:bool)
        "Boolean" <- w356
        n247 = case shown="True" w357 {
          frame False {
          }
          frame True {
            n248 = local write "Numeric 2"(0.0 ("Numeric 2")) -> ()
          }
        }
        n249 = case shown="False" w356 {
          frame False {
            n250 = property on="Lenguage" class="Bool (strict)"("BoolText.Text"="Español" ("Boolean Text.Text")) -> ()  [unwired: 2 in, 2 out]
          }
          frame True {
            n251 = property on="Lenguage" class="Bool (strict)"("BoolText.Text"="English" ("Boolean Text.Text")) -> ()  [unwired: 2 in, 2 out]
          }
        }
        n252 = call "MainEnQueue.vi"("States"=T6 {"States"=enum."Lenguaje", "Data"=variant}) -> ("error out"=w365:errorcluster)  [unwired: 10 in]
      }
      event "Help": Value Change {
        n253 = event-data() -> ()  [unwired: 1 in, 6 out]
      }
      event "Exit Button": Value Change {
        n254 = event-data() -> ()  [unwired: 1 in, 1 out]
        n255 = call "MainEnQueue.vi"("error in"=w369, "Array States"=T6[] [{"States"=enum."Close Ports", "Data"=variant}, {"States"=enum."Exit", "Data"=variant}]) -> ("error out"=w370:errorcluster)  [unwired: 9 in]
      }
      event Panel Close? {
        n256 = event-data() -> ()  [unwired: 1 in, 1 out]
        n257 = call "MainEnQueue.vi"("error in"=w373, "Array States"=T6[] [{"States"=enum."Close Ports", "Data"=variant}, {"States"=enum."Exit", "Data"=variant}]) -> ("error out"=w375:errorcluster)  [unwired: 9 in]
        n258 = event-data() -> ()  [unwired: 2 in, 1 out]
      }
      event "Cluster.24v": Value Change {
        n259 = event-data() -> ()  [unwired: 1 in, 1 out]
        n260 = local read "Sets"() -> (w384:T4)
        n261 = Bundle(cluster=w384, "String"="OUTP:COUP ACDC " ("String 1"), "String 2"="VOLT 0", "String 3"="VOLT:OFFS 22", "String 4"="VOLT:RANG MAX") -> (w385:T4)
        n262 = local write "Sets"(w385) -> ()
        n263 = Concatenate Strings("\r" ("Carriage Return Constant"), "24 Volts DC" ("Acción")) -> (w379:string)
        n264 = local write "Numeric"(24.0 ("Numeric")) -> ()
        n265 = property on="Acción" class="Str"("Value"=w379) -> ()  [unwired: 2 in, 2 out]
      }
      event "Cluster.48v": Value Change {
        n266 = event-data() -> ()  [unwired: 1 in, 6 out]
        n267 = local read "Sets"() -> (w394:T4)
        n268 = Concatenate Strings("\r" ("Carriage Return Constant"), "48 Volts DC" ("Acción")) -> (w389:string)
        n269 = property on="Acción" class="Str"("Value"=w389) -> ()  [unwired: 2 in, 2 out]
        n270 = Bundle(cluster=w394, "String"="OUTP:COUP ACDC " ("String 1"), "String 2"="VOLT 0", "String 3"="VOLT:OFFS 46", "String 4"="VOLT:RANG MAX") -> (w395:T4)
        n271 = local write "Sets"(w395) -> ()
        n272 = local write "Numeric"(48.0 ("Numeric")) -> ()
      }
      event "Cluster.110v": Value Change {
        n273 = event-data() -> ()  [unwired: 1 in, 6 out]
        n274 = local read "Sets"() -> (w404:T4)
        n275 = Concatenate Strings("\r" ("Carriage Return Constant"), "110 Volts AC" ("Acción")) -> (w399:string)
        n276 = Bundle(cluster=w404, "String"="OUTP:COUP ACDC " ("String 1"), "String 2"="VOLT 108", "String 3"="VOLT:OFFS 0", "String 4"="VOLT:RANG MAX") -> (w405:T4)
        n277 = property on="Acción" class="Str"("Value"=w399) -> ()  [unwired: 2 in, 2 out]
        n278 = local write "Numeric"(110.0 ("Numeric")) -> ()
        n279 = local write "Sets"(w405) -> ()
      }
      event "Cluster.220v": Value Change {
        n280 = event-data() -> ()  [unwired: 1 in, 6 out]
        n281 = Concatenate Strings("\r" ("Carriage Return Constant"), "220 Volts AC" ("Acción")) -> (w413:string)
        n282 = local read "Sets"() -> (w414:T4)
        n283 = property on="Acción" class="Str"("Value"=w413) -> ()  [unwired: 2 in, 2 out]
        n284 = Bundle(cluster=w414, "String"="OUTP:COUP ACDC " ("String 1"), "String 2"="VOLT 218", "String 3"="VOLT:OFFS 0", "String 4"="VOLT:RANG MAX") -> (w415:T4)
        n285 = local write "Sets"(w415) -> ()
        n286 = local write "Numeric"(220.0 ("Numeric")) -> ()
      }
      event "Cluster.OK Button Volts": Value Change {
        n287 = event-data() -> ()  [unwired: 1 in, 6 out]
        n288 = call "MainEnQueue.vi"("States"=T6 {"States"=enum."Volts", "Data"=variant}) -> ("error out"=w416:errorcluster)  [unwired: 10 in]
      }
      event "Cluster.Cancel Button Volts": Value Change {
        n289 = event-data() -> ()  [unwired: 1 in, 6 out]
        n290 = local read "Voltaje de salida"() -> (w418:dbl)
        n291 = local write "Numeric"(w418) -> ()
        n292 = call "MainEnQueue.vi"("States"=T6 {"States"=enum."Main", "Data"=variant}) -> ("error out"=w420:errorcluster)  [unwired: 10 in]
      }
      event "Start Test": Value Change {
        w422 = TRUE ("Visible")
        n293 = event-data() -> ()  [unwired: 1 in, 1 out]
        n294 = Wait (ms)(milliseconds to wait=u32 100) -> ()  [unwired: 1 out]
        n295 = property on="Start Time" class="Str"("Visible"=w422) -> ()  [unwired: 2 in, 2 out]
        n296 = property on="End Time" class="Str"("Visible"=w422) -> ()  [unwired: 2 in, 2 out]
        n297 = property on="Current Time" class="Str"("Visible"=w422) -> ()  [unwired: 2 in, 2 out]
        n298 = call "MainEnQueue.vi"("error in"=w423, "States"=T6 {"States"=enum."Test", "Data"=variant}) -> ("error out"=w424:errorcluster)  [unwired: 9 in]
      }
    }
  }
  n299 = for {
    N: 8 -> [_]
    tunnel: [u32 15263976] -> w4 mode=indexing
  }
  n300 = local write "Voltaje de salida"(0.0 ("Voltaje de salida")) -> ()
  n301 = local write "Cartuchos"(w4) -> ()
  n302 = disable-structure shown="Disabled" {
    frame Disabled {
      n303 = Format Into String(format string="%s\\r\\n", "VOLT:OFFS ?" ("data in")) -> (resulting string=w451:string)  [unwired: 2 in, 1 out]
      n304 = TCP Open Connection(address="169.254.73.86", remote port or service name=u16 5025, timeout ms (60000)=5000) -> (connection ID=w456:refnum<k5>, error out=w457:errorcluster)  [unwired: 2 in]
      n305 = call "TCP IP.vi"("String 4"="VOLT:OFFS 0", "String 3"="VOLT 0", "String 2"="OUTP OFF", "String 1"="OUTP:COUP ACDC") -> ()  [unwired: 1 out]
      n306 = TCP Write(connection ID=w456, data in=w451, error in (no error)=w457) -> (connection ID out=w450:refnum<k5>, bytes written=→"bytes written":i32, error out=w449:errorcluster)  [unwired: 1 in]
      n307 = TCP Read(connection ID=w450, bytes to read=500 ("timeout ms (25000)"), error in (no error)=w449, 7:T10."Buffered" ("mode (standard)")) -> (connection ID out=w447:refnum<k5>, data out=w443:string, error out=w448:errorcluster)  [unwired: 1 in]
      "data out" <- w443
      n308 = local read "Sets"() -> (w435:T4)
      n309 = TCP Close Connection(connection ID=w447, error in (no error)=w448) -> ()  [unwired: 1 in, 2 out]
      n310 = Fract/Exp String To Number(string=w443) -> (offset past number=→"offset past number":i32, number=→"number":dbl)  [unwired: 3 in]
      n311 = local read item#-1() -> (w438)
      n312 = Bundle(cluster=w435, "String"="OUTP:COUP ACDC " ("String 1"), "String 2"="VOLT 0", "String 3"="VOLT:OFFS 24", "String 4"="VOLT:RANG MAX") -> (w436:T4)
      n313 = local write "Sets"(w436) -> ()
      n314 = for {
        N: 10 -> [_]
        tunnel: [w459] -> w439 mode=indexing
        tunnel: w438 -> [w458]
        n315 = case shown="False" w458 {
          tunnel: [u32 16711680 u32 6291200] -> w459
          frame False {
          }
          frame True {
          }
        }
      }
      n316 = local write "Cartuchos"(w439) -> ()
    }
    frame Enabled {
    }
  }
  n317 = Merge Errors(w9, w8) -> (w7:errorcluster)
  n318 = disable-structure shown="Disabled" {
    disable-tunnel: w13 -> [w462 _]
    frame Disabled {
      n319 = Quit LabVIEW(quit? (T)=w462) -> ()
    }
    frame Enabled {
    }
  }
  n320 = property on="error out" class="Clust (strict)"(error in=w7, "Value"=w7) -> ()  [unwired: 1 in, 2 out]
  "Indicators" <- T8 {"Error Out Array"=[{"status"=FALSE, "code"=0, "source"=""}], "34970A"=FALSE, "53220A"=FALSE, "USB-CAN"=FALSE, "USB-LIN"=FALSE, "Voltage output"=TRUE} ("Indicators")
  "Acción" <- "" ("Acción")
  "0" <- cluster{i32, i32, i32, i32, i32, i32, i32, i32} {0, 1, 4, 5, 6, 7, 2, 3}
